vi "Tracer_Level-Generic.vi"(11 "Calltree Level":i32) -> (2 "Trace Enabled":bool, 3 "Category":string)   [LabVIEW 2018, in "TracerLibrary.lvlib" / "Tracer.lvclass"]
uses:
  Tracer.lvclass
  protected/Tracer_ClassAttributes.vi
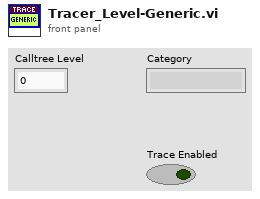
[diagram p1: front panel]
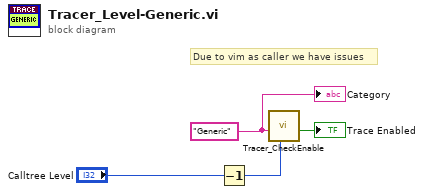
[diagram p0: block diagram]
diagram:
  w3 = "Generic" ("Category")
  # "Due to vim as caller we have issues"
  n1 = Decrement(x="Calltree Level") -> (x-1=w1:i32)
  n2 = call "Tracer_CheckEnable.vi"("Calltree Level"=w1, "Category"=w3) -> ("Trace Enabled"=→"Trace Enabled":bool)  [unwired: 9 in]
  "Category" <- w3
